vi "FlatToRichmicron_MessageRequest.vi"(5 "OutputClusterType":T1, 11 "InputCluster":T2) -> (3 "OutputCluster":T1)   [LabVIEW 2019, in "Micron_server.lvlib"]
uses:
  Micron_server.lvlib
  micron_MessageRequest_Flat.ctl
  micron_MessageRequest.ctl
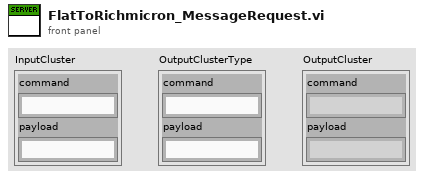
[diagram p1: front panel]
types:
  T1 = typedef "Micron_server.lvlib/micron_MessageRequest.ctl" = cluster{"command":string, "payload":string}
  T2 = typedef "Micron_server.lvlib/micron_MessageRequest_Flat.ctl" = cluster{"command":string, "payload":string}
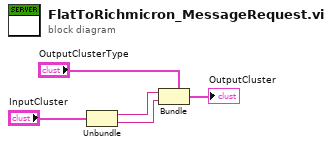
[diagram p0: block diagram]
diagram:
  n1 = Unbundle "Unbundle"("InputCluster") -> ("command"=w2:string, "payload"=w1:string)
  n2 = Bundle "Bundle"(cluster="OutputClusterType", "command"=w2, "payload"=w1) -> (→"OutputCluster":T1)
